vi "5492_ZeroYawCheck.vi"(8 "error in":errorcluster) -> (0 "error out":errorcluster)   [LabVIEW 2016]
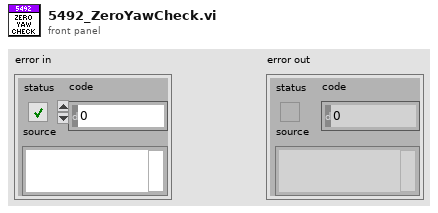
[diagram p1: front panel]
types:
  T1 = cluster{"Yaw":dbl, "Roll":dbl, "Pitch":dbl, "Heading":dbl, "Fused Heading":dbl}
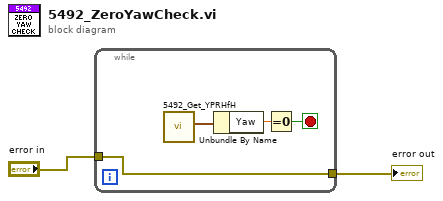
[diagram p0: block diagram]
diagram:
  n1 = while {
    tunnel: [w3] -> w2
    tunnel: "error in" -> [w3]
    stop <- w5 stop-if-true
    n2 = call "5492_Get_YPRHfH.vi"() -> ("YRPHfH"=w4:T1)  [unwired: 10 in, 1 out]
    n3 = Unbundle By Name(w4) -> ("Yaw"=w6:dbl)
    n4 = Equal To 0?(x=w6) -> (x = 0?=w5:bool)
  }
  "error out" <- w2
